vi "Configure Modulation (FSK).vi"(0 "VISA resource name":refnum<visa-resource-name>, 1 "Enable FSK Modulation (T: Enable)":bool=TRUE, 5 "Channel (1: Channel 1)":u16(ring)=1 items=["Channel 1"=1, "Channel 2"=2], 7 "FSK Modulation Source (0: Internal)":u16(ring) items=["Internal", "External"], 9 "Hop Frequency (100.00 Hz)":dbl=100.0 format="%.2f", 11 "error in (no error)":errorcluster, 12 "Internal Rate (100.00 Hz)":dbl=100.0 format="%.2f") -> (4 "VISA resource name out":refnum<visa-resource-name>, 15 "error out":errorcluster)   [LabVIEW 2016, in "Tektronix AFG 1000 Series.lvlib"]
doc: "Configures and enables Frequency-Shift Keying (FSK) modulation. The function generator shifts its output frequency between two present values."
uses:
  Tektronix AFG 1000 Series.lvlib
panel:
  # "Internal FSK Settings"
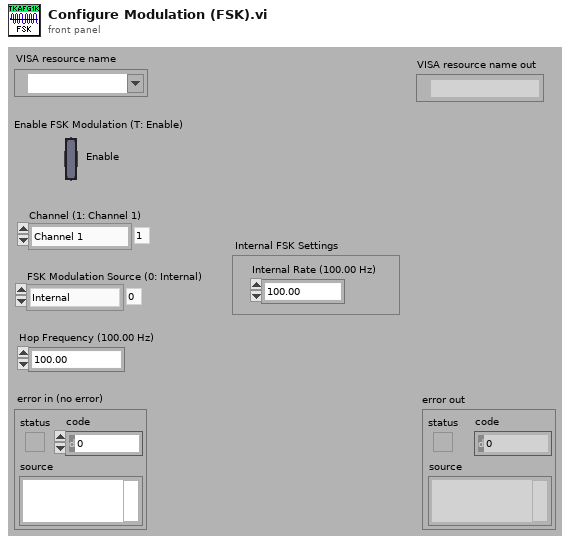
[diagram p1: front panel]
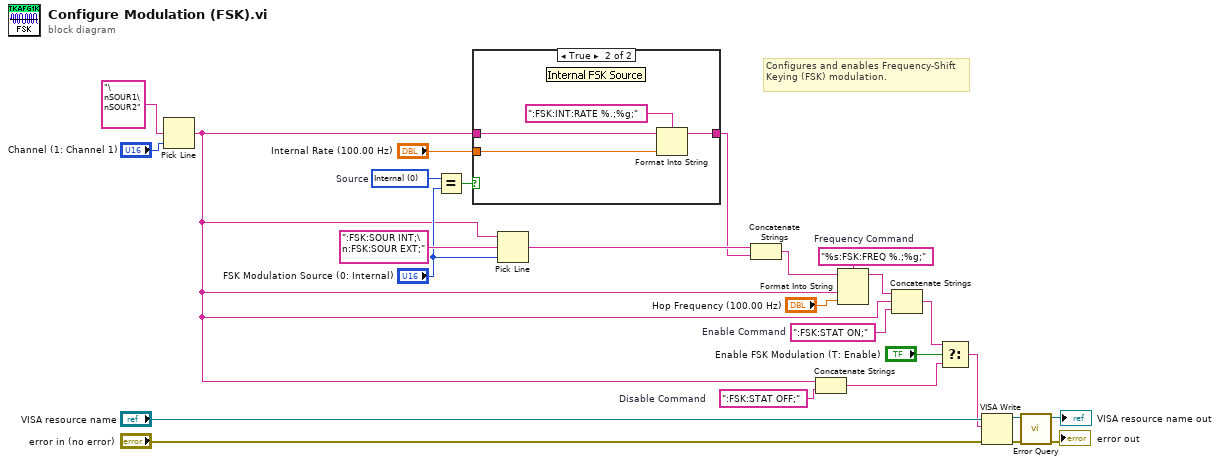
[diagram p0: block diagram]
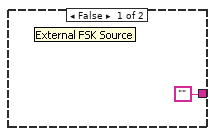
[diagram p2: hidden frame]
diagram:
  w19 = "%s:FSK:FREQ %.;%g;"  # Frequency Command
  w2 = ":FSK:STAT ON;"  # Enable Command
  w8 = u16 0 items=["Internal", "External"]  # Source
  w12 = ":FSK:STAT OFF;"  # Disable Command
  # "Configures and enables Frequency-Shift Keying (FSK) modulation."
  n1 = Pick Line(multi-line string="\nSOUR1\nSOUR2" ("string (\"\")"), line index="Channel (1: Channel 1)") -> (output string=w1:string)  [unwired: 1 in]
  n2 = Equal?(x=w8, y="FSK Modulation Source (0: Internal)") -> (x = y?=w10:bool)
  n3 = case shown="True" w10 {
    tunnel: ["" w30] -> w6
    tunnel: w1 -> [_ w29]
    tunnel: "Internal Rate (100.00 Hz)" -> [_ w28]
    frame False {
    }
    frame True {
      n4 = Format Into String(format string=":FSK:INT:RATE %.;%g;" ("initial string"), initial string=w29, w28) -> (resulting string=w30:string)  [unwired: 1 in, 1 out]
    }
  }
  n5 = Pick Line(string ("")=w1, multi-line string=":FSK:SOUR INT;\n:FSK:SOUR EXT;" ("string (\"\")"), line index="FSK Modulation Source (0: Internal)") -> (output string=w7:string)
  n6 = Concatenate Strings(w7, w6) -> (w5:string)
  n7 = Concatenate Strings(w1, w12) -> (w11:string)
  n8 = Format Into String(format string=w19, initial string=w5, w1, "Hop Frequency (100.00 Hz)") -> (resulting string=w20:string)  [unwired: 1 in, 1 out]
  n9 = Concatenate Strings(w20, w1, w2) -> (w13:string)
  n10 = Select(t=w13, s="Enable FSK Modulation (T: Enable)", f=w11) -> (s? t:f=w14:string)
  n11 = VISA Write(VISA resource name="VISA resource name", write buffer=w14, error in (no error)="error in (no error)") -> (VISA resource name out=w25:refnum<visa-resource-name>, error out=w24:errorcluster)  [unwired: 1 out]
  n12 = call "Error Query.vi"("error in (no error)"=w24, "VISA resource name"=w25) -> ("error out"=→"error out":errorcluster, "VISA resource name out"=→"VISA resource name out":refnum<visa-resource-name>)  [unwired: 6 in, 2 out]
